vi "Read Multi-Channel Waveform.vi"(8 "error in (no error)":errorcluster, 10 "Channels":T1[](array[typedef]), 11 "DPO4104 in":refnum<class "DPO4104.lvclass">) -> (0 "error out":errorcluster, 2 "Waveform":waveform(dbl)[](graph), 3 "DPO4104 out":refnum<class "DPO4104.lvclass">)   [LabVIEW 2018, in "DPO4104.lvlib" / "DPO4104.lvclass"]
doc: "This Override method is used to initiate multi-channel waveform acquisition. Select targeted channels at the 'Channels' control and output waveform data to the 'Waveform' indicator."
uses:
  DPO4104.lvclass
  PPLs/Oscilloscope/Parent/Oscilloscope.lvlibp/Custom Controls/Analog Channels.ctl
  PPLs/Oscilloscope/Parent/Oscilloscope.lvlibp/Oscilloscope.lvclass
  <instrlib>/Tektronix DPO MSO 2000 4000 Series/Tektronix DPO MSO 2000 4000 Series.lvlib
  C:/Projects/LabVIEW/PPLs/Oscilloscope/Parent/Oscilloscope.lvlibp/Oscilloscope.lvclass
  PPLs/Oscilloscope/Parent/Oscilloscope.lvlibp
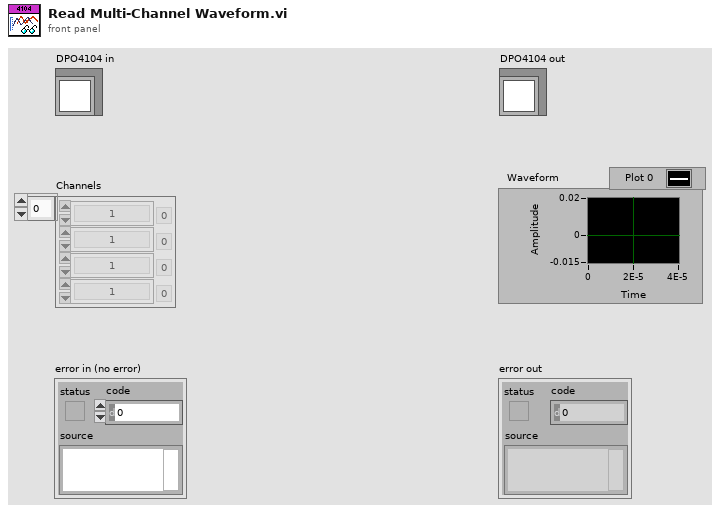
[diagram p1: front panel]
types:
  T1 = typedef "Oscilloscope.lvlibp/Analog Channels.ctl" = enum16{"1", "2", "3", "4", "5", "6", "7", "8", "9", "10", "11", "12", "13", "14", "15", "16"}
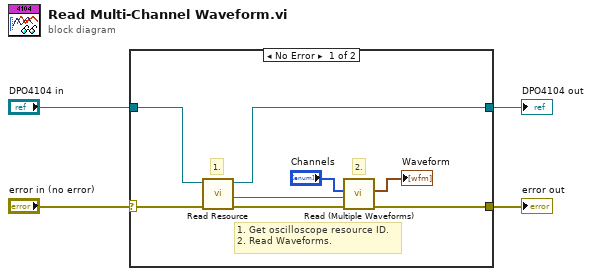
[diagram p0: block diagram]
diagram:
  n1 = case shown="No Error" "error in (no error)" {
    selector: "error in (no error)" -> [w10 w13]
    tunnel: [w7 w13] -> w3
    tunnel: [w11 w14] -> w2
    tunnel: "DPO4104 in" -> [w12 w14]
    frame No Error {
      # "2."
      # "1."
      # "1. Get oscilloscope resource ID.\n2. Read Waveforms."
      n2 = call "Read Resource.vi"("error in (no error)"=w10, "Oscilloscope in"=w12) -> ("error out"=w8:errorcluster, "Resource"=w9:refnum<visa-resource-name>, "Oscilloscope out"=w11:refnum<class "DPO4104.lvclass">)  [unwired: 7 in]
      n3 = call <instrlib>:"Read (Multiple Waveforms).vi"("error in (no error)"=w8, "Channels"="Channels", "VISA resource name"=w9) -> ("error out"=w7:errorcluster, "Waveform Data"=→"Waveform":waveform(dbl)[])  [unwired: 6 in, 1 out]
    }
    frame Error {
    }
  }
  "error out" <- w3
  "DPO4104 out" <- w2
